vi "open v2.vi"(7 "zVfs":i32, 8 "error in (no error)":errorcluster, 9 "custom flags(rw/create)":i32 format="%x", 11 "filename":path) -> (0 "error out":errorcluster, 2 "ppDb out":u64)   [LabVIEW 2020, in "sqlite3.lvlib"]
uses:
  sqlite3.lvlib
  errstr.vi
  bin/sqlite3_64.dll
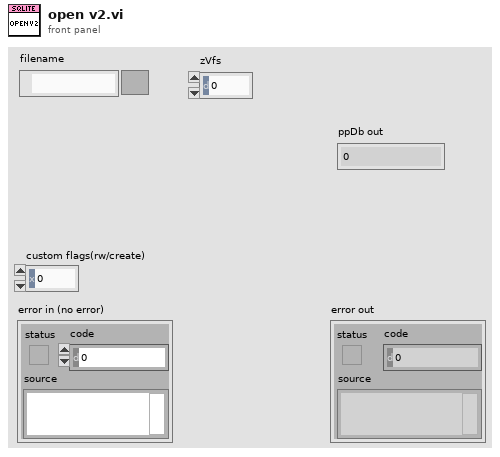
[diagram p1: front panel]
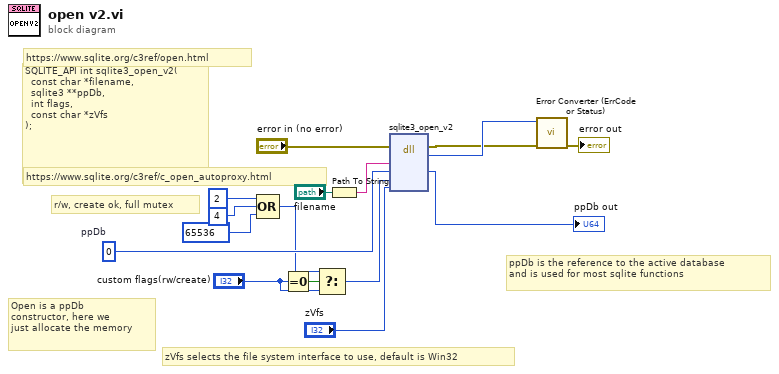
[diagram p0: block diagram]
diagram:
  w14 = u64 0  # ppDb
  # "zVfs selects the file system interface to use, default is Win32"
  # "ppDb is the reference to the active database\nand is used for most sqlite functions"
  # "r/w, create ok, full mutex"
  # "Open is a ppDb\nconstructor, here we \njust allocate the memory"
  # "https://www.sqlite.org/c3ref/open.html"
  # "https://www.sqlite.org/c3ref/c_open_autoproxy.html"
  # "SQLITE_API int sqlite3_open_v2(\n  const char *filename,   \n  sqlite3 **ppDb,         \n  int flags,              \n  const char *zVfs        \n);"
  n1 = Compound Arithmetic op=OR(2 ("value"), 4 ("value"), 65536 ("value")) -> (w5:i32)
  n2 = Equal To 0?(x="custom flags(rw/create)") -> (x = 0?=w9:bool)
  n3 = Select(t=w5, s=w9, f="custom flags(rw/create)") -> (s? t:f=w8:i32)
  n4 = Path To String(path="filename") -> (string=w2:string)
  n5 = dll-call lib="D:/Project/Labview-Projects/database-configuration/externals/sqlite3/Source/bin/sqlite3_*.*" fn="sqlite3_open_v2"(error in="error in (no error)", "filename"=w2, "ppDb"=w14, "flags"=w8, "zVfs"="zVfs") -> (error out=w11:errorcluster, "return type"=w16:i32, "ppDb"=→"ppDb out":u64)  [unwired: 5 in, 1 out]
  n6 = call "Error Converter (ErrCode or Status).vi"("error in (no error)"=w11, "error code"=w16) -> ("error out"=→"error out":errorcluster)  [unwired: 9 in]
